vi "Error Log GUI.vi"(6 "File Options":T1(ring)=enum."Read File", 8 "error in (no error)":errorcluster, 10 "Write":string, 11 "Post Analysis in":refnum<class "Post Analysis.lvclass">) -> (0 "error out":errorcluster, 3 "Post Analysis out":refnum<class "Post Analysis.lvclass">)   [LabVIEW 2023, in "Data Analysis.lvlib" / "Post Analysis.lvlib" / "Post Analysis.lvclass"]
uses:
  Post Analysis.lvclass
  Post Analysis.lvclass/Post Analysis.ctl
panel:
  out "Read":string
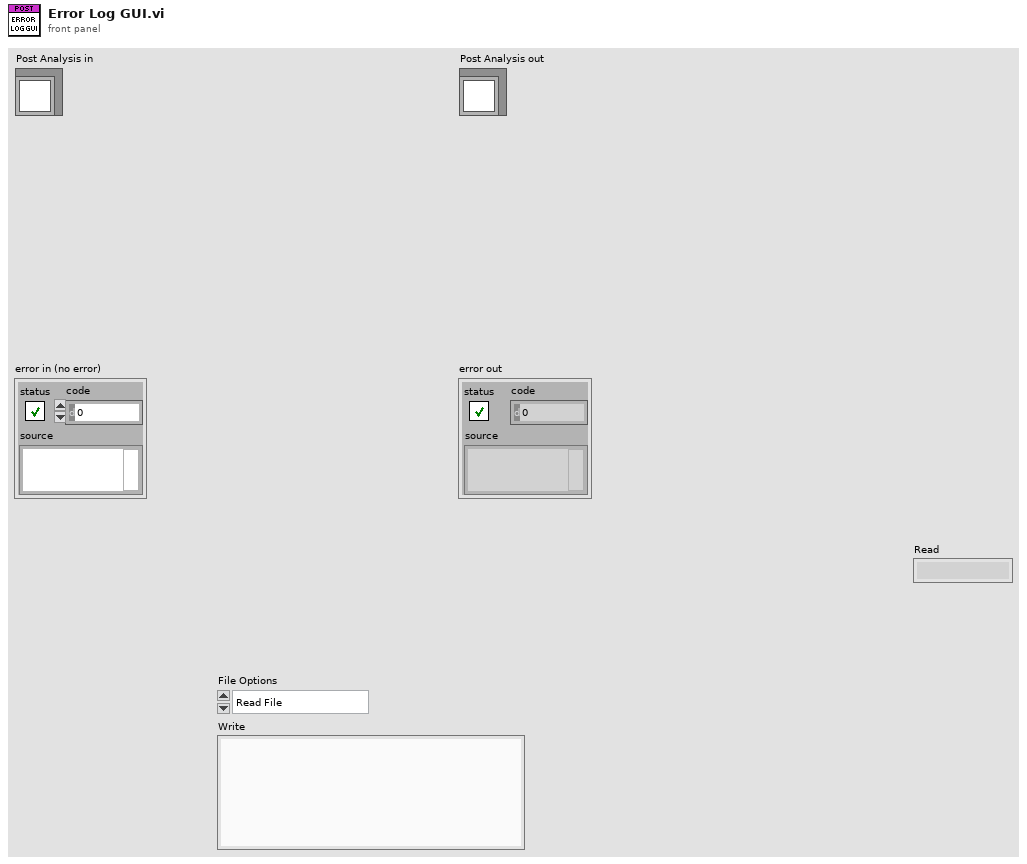
[diagram p1: front panel]
types:
  T1 = enum16{"Open", "Read File", "Write File", "Close"}
  T2 = enum16{"open", "replace", "create", "open or create", "replace or create", "replace or create with confirmation"}
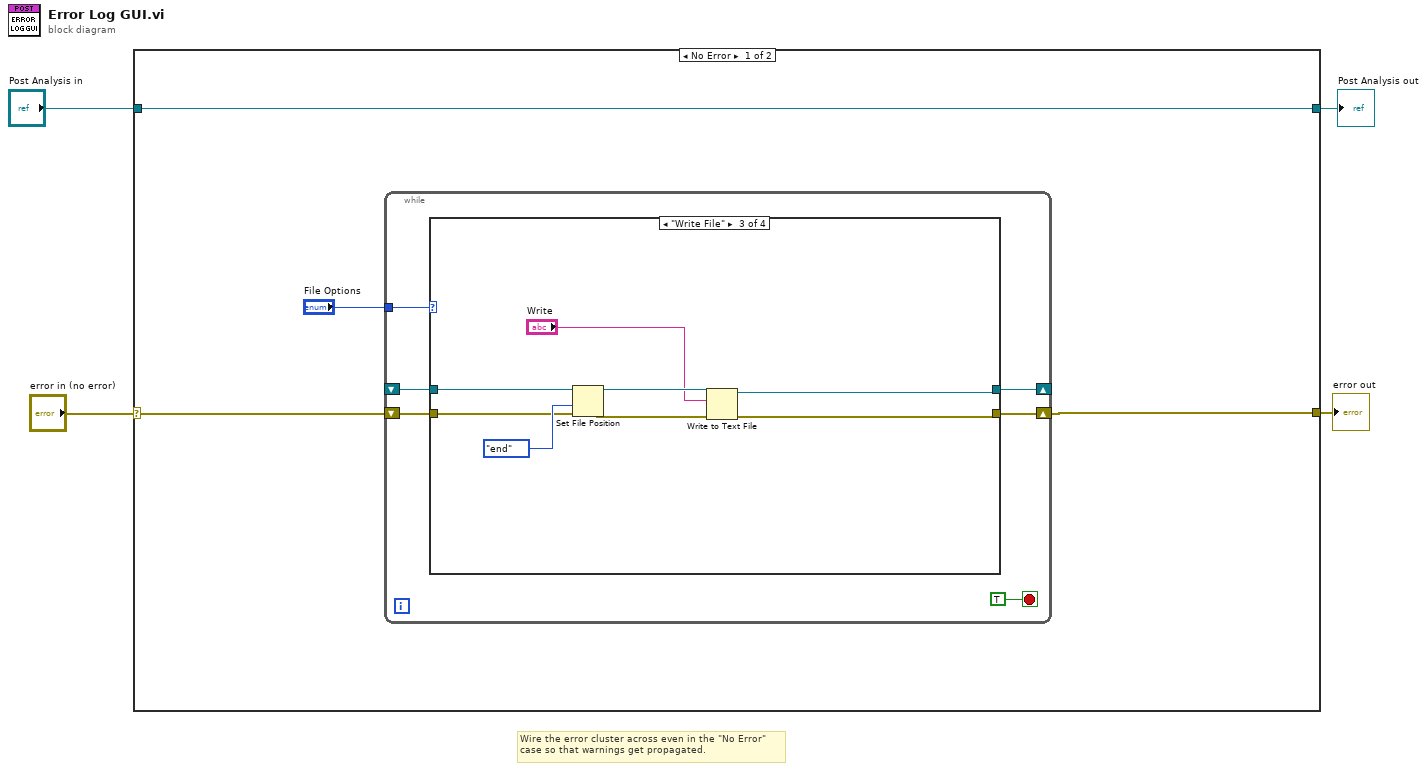
[diagram p0: block diagram]
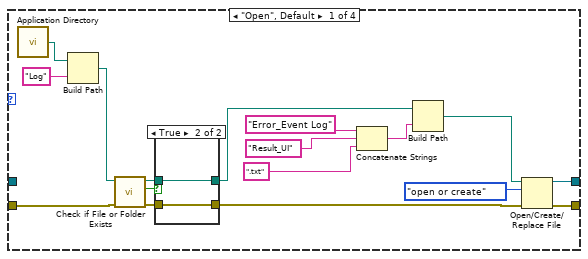
[diagram p2: hidden frame]
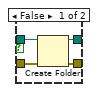
[diagram p3: hidden frame]
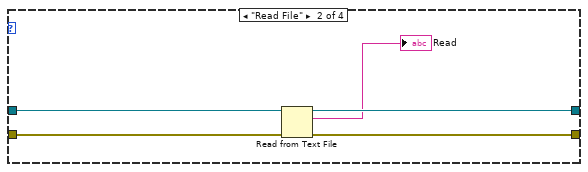
[diagram p4: hidden frame]
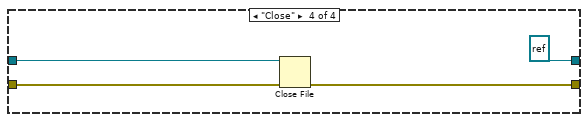
[diagram p5: hidden frame]
diagram:
  # "Wire the error cluster across even in the \"No Error\"\ncase so that warnings get propagated."
  n1 = case shown="No Error" "error in (no error)" {
    selector: "error in (no error)" -> [w5 w56]
    tunnel: [w6 w56] -> w3
    tunnel: [w8 w55] -> w1
    tunnel: "Post Analysis in" -> [w8 w55]
    frame No Error {
      n2 = while {
        tunnel: "File Options" -> [w14]
        shift-right: [w10] -> _
        shift-left: _ -> [w13]
        shift-right: [w11] -> w6
        shift-left: w5 -> [w12]
        stop <- TRUE stop-if-true
        n3 = case shown="\"Write File\"" w14 {
          tunnel: w13 -> [_ w42 w46 w52]
          tunnel: w12 -> [w17 w41 w47 w54]
          tunnel: [w23 w40 w50 w53] -> w11
          tunnel: [w22 w39 w49 refnum<file> refnum ("refnum out")] -> w10
          frame "Open", Default {
            n4 = call <vilib>:"Application Directory.vi"() -> ("Application Directory"=w24:path)
            n5 = Build Path(base path=w24, name or relative path="Log") -> (appended path=w21:path)
            n6 = call <vilib>:"Check if File or Folder Exists.vi"("error in (no error)"=w17, "path"=w21) -> ("error out"=w20:errorcluster, "file or folder exists?"=w15:bool, "dup path"=w19:path)  [unwired: 7 in]
            n7 = case shown="True" w15 {
              tunnel: w20 -> [w35 w36]
              tunnel: w19 -> [w34 w37]
              tunnel: [w33 w37] -> w18
              tunnel: [w32 w36] -> w16
              frame False {
                n8 = Create Folder(path (use dialog)=w34, error in=w35) -> (created path=w33:path, error out=w32:errorcluster)  [unwired: 1 in, 1 out]
              }
              frame True {
              }
            }
            n9 = Concatenate Strings("Error_Event Log", "Result_UI" ("File Name"), ".txt" ("string")) -> (w28:string)
            n10 = Build Path(base path=w18, name or relative path=w28) -> (appended path=w30:path)
            n11 = Open/Create/Replace File(file path (use dialog)=w30, error in=w16, operation (0:open)=T2."open or create") -> (refnum out=w22:refnum<file>, error out=w23:errorcluster)  [unwired: 3 in, 1 out]
          }
          frame "Read File" {
            n12 = Read from Text File(file (use dialog)=w42, error in=w41) -> (refnum out=w39:refnum<file>, text=→"Read":string, error out=w40:errorcluster)  [unwired: 2 in, 1 out]
          }
          frame "Write File" {
            n13 = Set File Position(refnum=w46, from (0:start)=enum16{"start", "end", "current"}."end", error in=w47) -> (refnum out=w45:refnum<file>, error out=w44:errorcluster)  [unwired: 1 in]
            n14 = Write to Text File(file (use dialog)=w45, text="Write", error in=w44) -> (refnum out=w49:refnum<file>, error out=w50:errorcluster)  [unwired: 1 in, 1 out]
          }
          frame "Close" {
            n15 = Close File(refnum=w52, error in=w54) -> (error out=w53:errorcluster)  [unwired: 1 out]
          }
        }
      }
    }
    frame Error {
    }
  }
  "error out" <- w3
  "Post Analysis out" <- w1
